vi "流量计参数设置.vi"(11 "MB session in":refnum<class "MB_Master.lvclass">) -> ()   [LabVIEW 2016, in "斯坦道功率测流.lvlib"]
uses:
  <vilib>/Plasmionique/MB Master/MB_Master/MB_Master.lvclass
panel:
  in  "关闭":bool
  out "状态值":T1
  in  "累积流量清零":bool
  in  "6号机组":bool
  in  "5号机组":bool
  in  "4号机组":bool
  in  "3号机组":bool
  in  "2号机组":bool
  in  "1号机组":bool
  out "水泵效率":dbl
  out "工质密度":dbl
  out "重力加速度":dbl
  out "水泵流量":dbl
  out "水泵扬程":dbl
  out "电机功率":dbl
  in  "Slave ID":u8(ring)=20 items=["1#测流计"=20, "2#测流计"=21]
  # "斯坦道功率测流参数设置"
  # "N=Q.H.g.ρ /η\nN——电机功率，kW\nH——水泵扬程，m\nQ——水泵流量，m^3/s\ng——重力加速度g=9.81\nρ ——工质的密度，当工质是水时，ρ=1\nη——水泵效率，查不到数值时可取η=0.8"
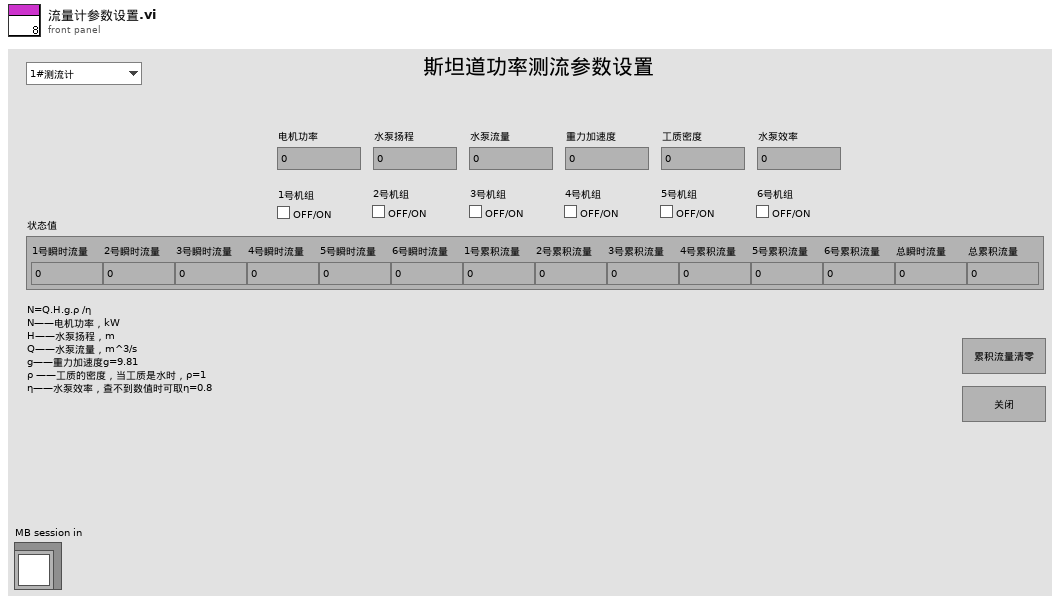
[diagram p1: front panel]
types:
  T1 = typedef "斯坦道功率测流.lvlib/状态值.ctl" = cluster{"1号瞬时流量":dbl, "2号瞬时流量":dbl, "3号瞬时流量":dbl, "4号瞬时流量":dbl, "5号瞬时流量":dbl, "6号瞬时流量":dbl, "1号累积流量":dbl, "2号累积流量":dbl, "3号累积流量":dbl, "4号累积流量":dbl, "5号累积流量":dbl, "6号累积流量":dbl, "总瞬时流量":dbl, "总累积流量":dbl}
  T2 = typedef "斯坦道功率测流.lvlib/测流参数.ctl" = cluster{"电机功率":dbl, "水泵扬程":dbl, "水泵流量":dbl, "重力加速度":dbl, "工质密度":dbl, "水泵效率":dbl, "流量计1启用":u16, "流量计2启用":u16, "流量计3启用":u16, "流量计4启用":u16, "流量计5启用":u16, "流量计6启用":u16, "累积流量清零":u16}
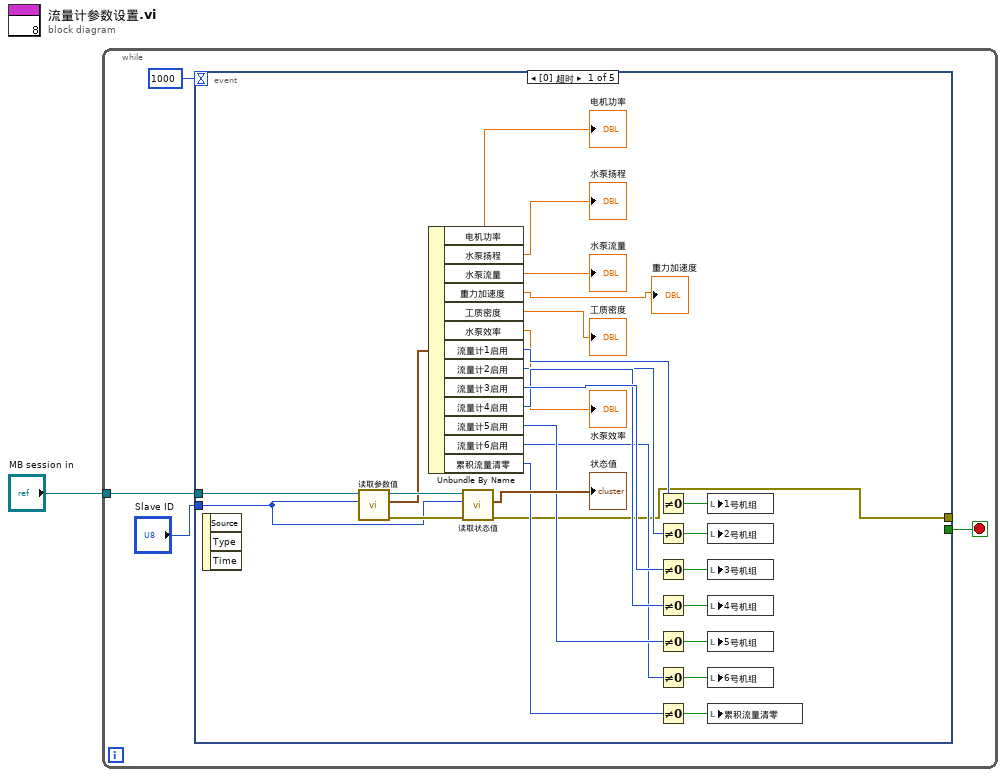
[diagram p0: block diagram]
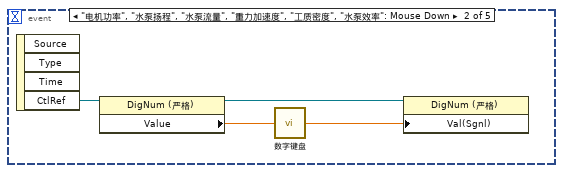
[diagram p2: hidden frame]
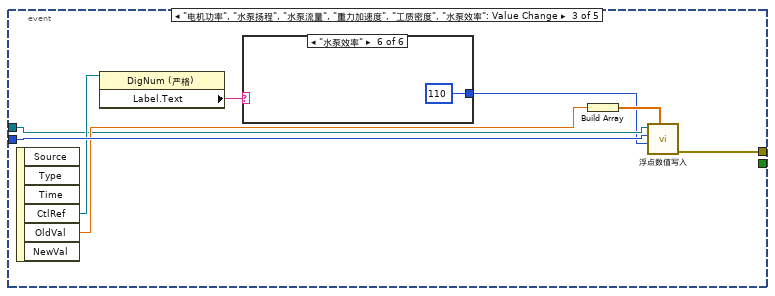
[diagram p3: hidden frame]
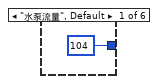
[diagram p4: hidden frame]
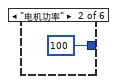
[diagram p5: hidden frame]
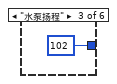
[diagram p6: hidden frame]
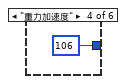
[diagram p7: hidden frame]
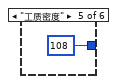
[diagram p8: hidden frame]
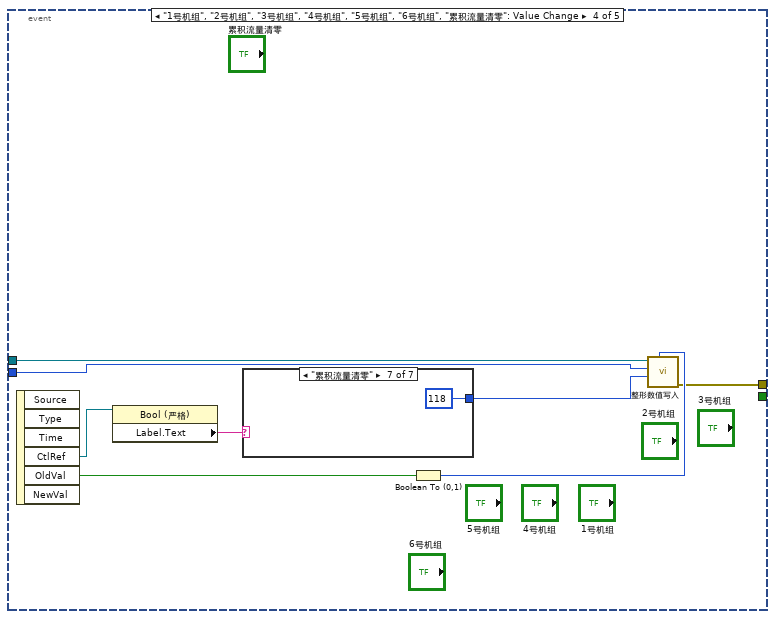
[diagram p9: hidden frame]
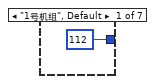
[diagram p10: hidden frame]
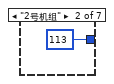
[diagram p11: hidden frame]
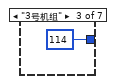
[diagram p12: hidden frame]
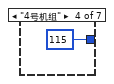
[diagram p13: hidden frame]
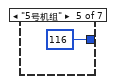
[diagram p14: hidden frame]
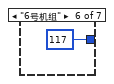
[diagram p15: hidden frame]
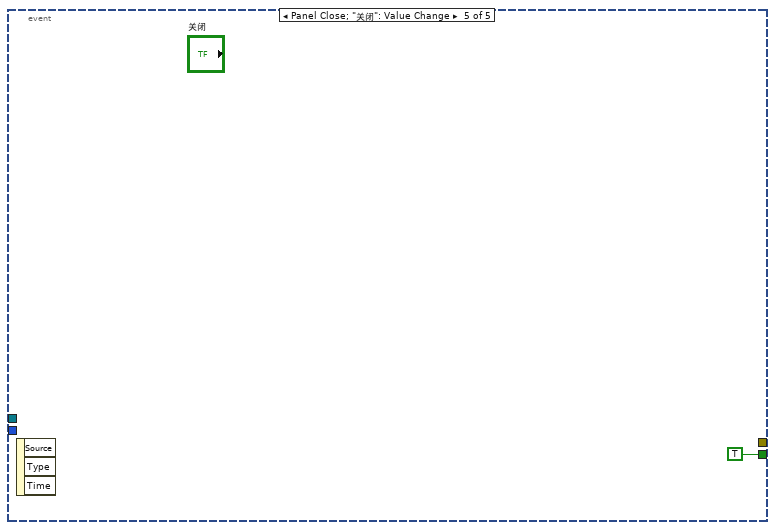
[diagram p16: hidden frame]
diagram:
  n1 = while {
    tunnel: "MB session in" -> [w4]
    stop <- w3 stop-if-true
    n2 = event shown="[0] 超时" {
      selector: _ -> [_ _ _ _ _]
      dyn-events: _ -> [_ _ _ _ _]
      timeout: 1000 -> [_ _ _ _ _]
      tunnel: w4 -> [w32 _ w39 w56 _]
      tunnel: [_ _ _ _ TRUE] -> w3
      tunnel: "Slave ID" -> [w7 _ w44 w55 _]
      tunnel: [w6 _ w37 w51 _] -> _
      event Timeout {
        n3 = event-data() -> ()  [unwired: 1 in, 3 out]
        n4 = call "读取参数值.vi"("Slave ID"=w7, "MB session in"=w32) -> ("error out"=w31:errorcluster, "测流参数"=w28:T2, "MB session out"=w30:refnum<class "MB_Master.lvclass">)  [unwired: 6 in, 1 out]
        n5 = Unbundle By Name(w28) -> ("电机功率"=→"电机功率":dbl, "水泵扬程"=→"水泵扬程":dbl, "水泵流量"=→"水泵流量":dbl, "重力加速度"=→"重力加速度":dbl, "工质密度"=→"工质密度":dbl, "水泵效率"=→"水泵效率":dbl, "流量计1启用"=w27:u16, "流量计2启用"=w21:u16, "流量计3启用"=w25:u16, "流量计4启用"=w24:u16, "流量计5启用"=w23:u16, "流量计6启用"=w22:u16, "累积流量清零"=w20:u16)
        n6 = call "读取状态值.vi"("error in (no error)"=w31, "Slave ID"=w7, "MB session in"=w30) -> ("error out"=w6:errorcluster, "状态值"=→"状态值":T1)  [unwired: 5 in, 2 out]
        n7 = Not Equal To 0?(x=w27) -> (x != 0?=w26:bool)
        n8 = Not Equal To 0?(x=w21) -> (x != 0?=w19:bool)
        n9 = Not Equal To 0?(x=w25) -> (x != 0?=w18:bool)
        n10 = Not Equal To 0?(x=w24) -> (x != 0?=w17:bool)
        n11 = Not Equal To 0?(x=w23) -> (x != 0?=w16:bool)
        n12 = Not Equal To 0?(x=w22) -> (x != 0?=w15:bool)
        n13 = Not Equal To 0?(x=w20) -> (x != 0?=w14:bool)
        n14 = local write "1号机组"(w26) -> ()
        n15 = local write "2号机组"(w19) -> ()
        n16 = local write "3号机组"(w18) -> ()
        n17 = local write "4号机组"(w17) -> ()
        n18 = local write "5号机组"(w16) -> ()
        n19 = local write "6号机组"(w15) -> ()
        n20 = local write "累积流量清零"(w14) -> ()
      }
      event "电机功率", "水泵扬程", "水泵流量", "重力加速度", "工质密度", "水泵效率": Mouse Down {
        n21 = event-data() -> ("CtlRef"=w36:refnum<vi>)  [unwired: 1 in, 3 out]
        n22 = property class="DigNum (严格)"(reference=w36) -> (reference out=w33:refnum<vi>, "Value"=w35:dbl)  [unwired: 1 in, 1 out]
        n23 = call "数字键盘.vi"("OldNumber"=w35) -> ("NewNumber"=w34:sgl)
        n24 = property class="DigNum (严格)"(reference=w33, "Val(Sgnl)"=w34) -> ()  [unwired: 1 in, 2 out]
      }
      event "电机功率", "水泵扬程", "水泵流量", "重力加速度", "工质密度", "水泵效率": Value Change {
        n25 = event-data() -> ("CtlRef"=w43:refnum<vi>, "OldVal"=w41:dbl)  [unwired: 1 in, 4 out]
        n26 = property class="DigNum (严格)"(reference=w43) -> ("Label.Text"=w42:string)  [unwired: 1 in, 2 out]
        n27 = case shown="\"水泵效率\"" w42 {
          tunnel: [u16 104 ("starting address") u16 100 ("starting address") u16 102 ("starting address") u16 106 ("starting address") u16 108 ("starting address") u16 110 ("starting address")] -> w38
          frame "水泵流量", Default {
          }
          frame "电机功率" {
          }
          frame "水泵扬程" {
          }
          frame "重力加速度" {
          }
          frame "工质密度" {
          }
          frame "水泵效率" {
          }
        }
        n28 = Build Array(w41) -> (w40:dbl[])
        n29 = call "浮点数值写入.vi"("浮点"=w40, "starting address"=w38, "Slave ID"=w44, "MB session in"=w39) -> ("error out"=w37:errorcluster)  [unwired: 6 in, 1 out]
      }
      event "1号机组", "2号机组", "3号机组", "4号机组", "5号机组", "6号机组", "累积流量清零": Value Change {
        n30 = event-data() -> ("CtlRef"=w58:refnum<vi>, "OldVal"=w54:bool)  [unwired: 1 in, 4 out]
        n31 = property class="Bool (严格)"(reference=w58) -> ("Label.Text"=w57:string)  [unwired: 1 in, 2 out]
        n32 = case shown="\"累积流量清零\"" w57 {
          tunnel: [u16 112 ("starting address") u16 113 ("starting address") u16 114 ("starting address") u16 115 ("starting address") u16 116 ("starting address") u16 117 ("starting address") u16 118 ("starting address")] -> w52
          frame "1号机组", Default {
          }
          frame "2号机组" {
          }
          frame "3号机组" {
          }
          frame "4号机组" {
          }
          frame "5号机组" {
          }
          frame "6号机组" {
          }
          frame "累积流量清零" {
          }
        }
        n33 = Boolean To (0,1)(Boolean=w54) -> (0, 1=w53:i16)
        n34 = call "整形数值写入.vi"("value"=w53, "starting address"=w52, "Slave ID"=w55, "MB session in"=w56) -> ("error out"=w51:errorcluster)  [unwired: 6 in, 1 out]
      }
      event Panel Close; "关闭": Value Change {
        n35 = event-data() -> ()  [unwired: 1 in, 3 out]
      }
    }
  }
